vi "Command (write) - SI.vi"(7 "timeout ms (100)":i32=100, 8 "error in (no error)":errorcluster, 9 "Input Usage State":string, 10 "IP":string, 11 "connection ID in":refnum<k16>) -> (0 "error out":errorcluster, 3 "connection ID out":refnum<k16>)   [LabVIEW 2016, in "SMD-7615.lvlib" / "eSCL.lvlib"]
doc: "SI - Enable Input Usage\nSets or requests the usage of the Enable input. Input X3 is the default Enable input on all drives, however IN3 on SE, QE and Si drives may also be designated as the Enable input (see below). If an external Enable function is not needed input X3 and/or IN3 can be defined solely as a general purpose input. In this scenario only the ME and MD commands will enable and disable the drive, respectively. When using the brake output (see BO, BD and BE commands) the disabling of the drive is delayed by the time value set using the BD command.\n\nSI1: Drive is enabled when X3 is open (inactive, high).\nSI2: Drive is enabled when X3 is closed (active, low).\nSI3: Neither X3 nor IN3 is used for enabling/disabling the drive, but as general purpose inputs.\nSI4: Drive is enabled when IN3 is open (inactive, high). (SE, QE, and Si drives only).\nSI5: Drive is enabled when IN3 is closed (active, low). (SE, QE, and Si drives only)."
uses:
  eSCL.lvlib
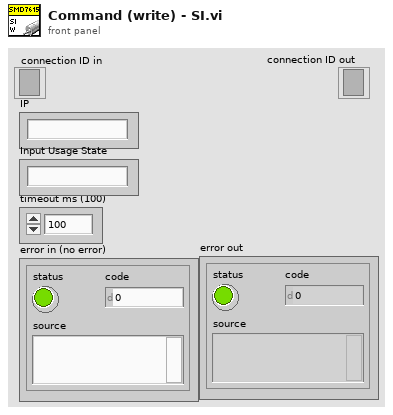
[diagram p1: front panel]
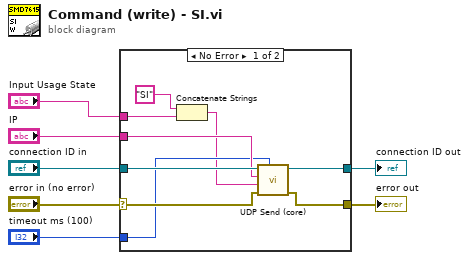
[diagram p0: block diagram]
diagram:
  n1 = case shown="No Error" "error in (no error)" {
    selector: "error in (no error)" -> [w16 w17]
    tunnel: "connection ID in" -> [w15 w18]
    tunnel: [w10 w18] -> w5
    tunnel: [w9 w17] -> w4
    tunnel: "IP" -> [w14 _]
    tunnel: "timeout ms (100)" -> [w13 _]
    tunnel: "Input Usage State" -> [w11 _]
    frame No Error {
      n2 = Concatenate Strings("SI" ("Data"), w11) -> (w8:string)
      n3 = call "UDP Send (core).vi"("timeout ms (100)"=w13, "error in (no error)"=w16, "Data"=w8, "IP"=w14, "connection ID in"=w15) -> ("error out"=w9:errorcluster, "connection ID out"=w10:refnum<k16>)  [unwired: 5 in]
    }
    frame Error {
    }
  }
  "connection ID out" <- w5
  "error out" <- w4
